vi "LED_LabView-RP2040.vi"() -> ()   [LabVIEW 2023]
uses:
  <vilib>/Instr/_visa.llb/VISA Configure Serial Port (Instr).vi
panel:
  in  "stop":bool
  out "String":string
  in  "VISA resource name":refnum<visa-resource-name>
  in  "Boolean":bool
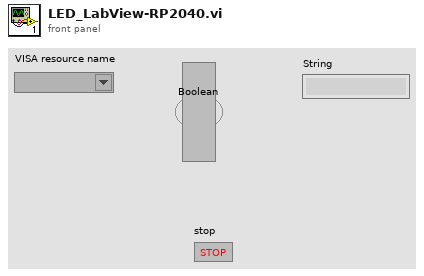
[diagram p1: front panel]
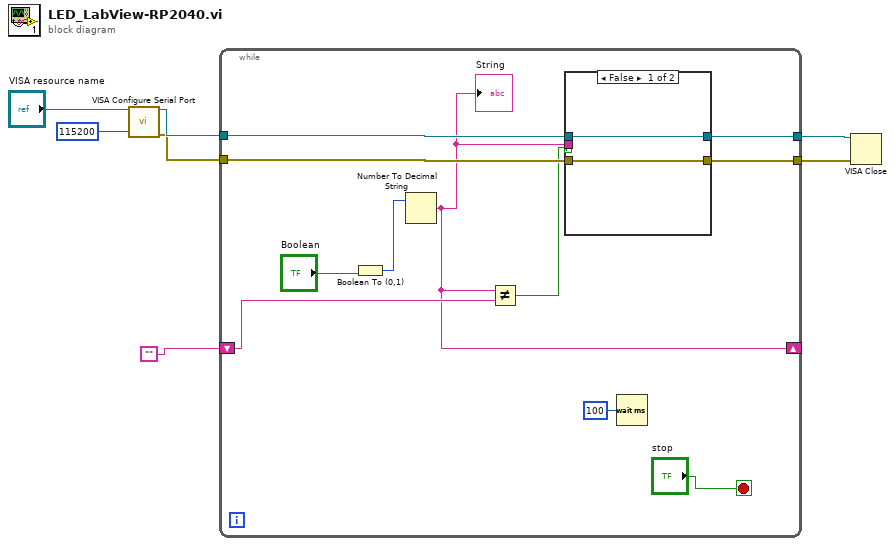
[diagram p0: block diagram]
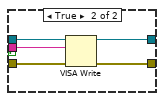
[diagram p2: hidden frame]
diagram:
  n1 = call-poly "VISA Configure Serial Port"("VISA resource name"="VISA resource name", "baud rate (9600)"=u32 115200) -> ("VISA resource name out"=w5:refnum<visa-resource-name>, "error out"=w4:errorcluster)  [unwired: 12 in]
  n2 = while {
    tunnel: w5 -> [w18]
    tunnel: w4 -> [w17]
    shift-right: [w9] -> _
    shift-left: "" -> [w10]
    tunnel: [w12] -> w3
    tunnel: [w11] -> w2
    stop <- "stop" stop-if-true
    n3 = Boolean To (0,1)(Boolean="Boolean") -> (0, 1=w15:i16)
    n4 = Number To Decimal String(number=w15) -> (decimal integer string=w9:string)  [unwired: 1 in]
    "String" <- w9
    n5 = Not Equal?(x=w9, y=w10) -> (x != y?=w8:bool)
    n6 = case shown="False" w8 {
      tunnel: w18 -> [w20 w25]
      tunnel: w17 -> [w19 w24]
      tunnel: w9 -> [_ w23]
      tunnel: [w20 w22] -> w12
      tunnel: [w19 w21] -> w11
      frame False {
      }
      frame True {
        n7 = VISA Write(VISA resource name=w25, write buffer=w23, error in (no error)=w24) -> (VISA resource name out=w22:refnum<visa-resource-name>, error out=w21:errorcluster)  [unwired: 1 out]
      }
    }
    n8 = Wait (ms)(milliseconds to wait=u32 100) -> ()  [unwired: 1 out]
  }
  n9 = VISA Close(VISA resource name=w3, error in (no error)=w2) -> ()  [unwired: 1 out]
